vi "Get density continuous samples to func glob PN.vi"(0 "Timing SW trigger":tag="Dev1/port2/line7", 1 "Counter":tag="Dev1/ctr0", 2 "Device":tag="Dev1") -> ()   [LabVIEW 2011]
uses:
  <vilib>/Platform/TimedLoop/XDataNode/timing_clust.ctl
  <vilib>/Platform/TimedLoop/XDataNode/nitl_modes.ctl
  <vilib>/Platform/TimedLoop/XDataNode/wakeup.ctl
  <vilib>/DAQmx/read.llb/DAQmx Read (Digital Bool 1Line 1Point).vi
  <vilib>/DAQmx/read.llb/DAQmx Read (Counter U32 1Chan 1Samp).vi
  <vilib>/DAQmx/create/channels.llb/DAQmx Create Channel (DI-Digital Input).vi
  <vilib>/DAQmx/create/channels.llb/DAQmx Create Channel (CI-Count Edges).vi
  <vilib>/DAQmx/miscellaneous.llb/DAQmx Fill In Error Info.vi
  <vilib>/Platform/TimedLoop/XDataNode/XDataNode.xnode
  <vilib>/Platform/TimedLoop/XDataNode/XDNodeRunTimeDep.lvlib
panel:
  out "Density (kg/m^3)":dbl
  out "Sample DateTime":timestamp
  out "current sample":i32
  out "Density history":u32(graph)=997
  in  "stop":bool
  out "reset state":bool
  out "Error":errorcluster
  # "by Paul Nathan,06/03/2012"
  # "Revisions:\nDate       Desc.      Auth.\nx               x               x"
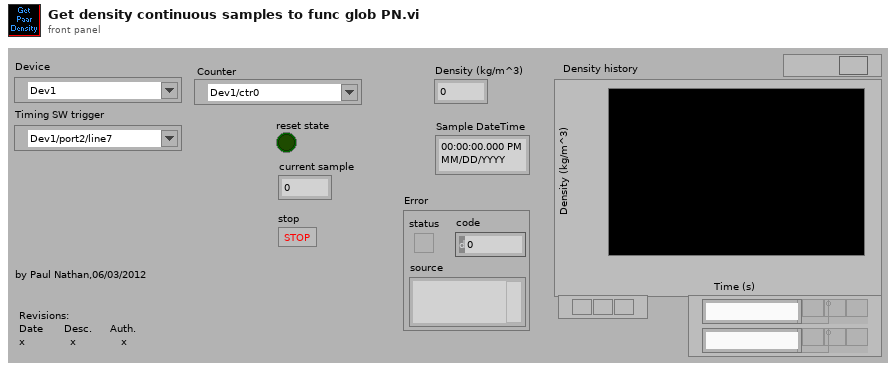
[diagram p1: front panel]
types:
  T1 = typedef "XDNodeRunTimeDep.lvlib/timing_clust.ctl" = cluster{"Expected End [f-1]":u64, "Actual End [f-1]":u64, "Finished Late? [f-1]":bool, "Expected End [i-1]":u64, "Actual End [i-1]":u64, "Finished Late? [i-1]":bool, "Expected Start [i]":u64, "Actual Start [i]":u64, "Expected Start [f]":u64, "Actual Start [f]":u64, "Source Name":string, "Structure Name":string, "Period":i64, "Deadline":i64, "Offset":i64, "Start":i64, "Priority":i32, "Timeout":i32, "Mode":T2, "Wakeup Reason":T3, "Error":errorcluster, "Source Type":string, "Secondary Source Type":string, "Global End Time":u64, "Global Start Time":u64, "Frame Duration":u64, "Iteration Duration":u64, "Assigned CPU":i32, "I/O Scan Engine Mode":u32}
  T2 = typedef "XDNodeRunTimeDep.lvlib/nitl_modes.ctl" = enum32{"No Change", "Process missed periods, maintain original phase", "Discard missed periods, maintain original phase", "Process missed periods, ignore original phase", "Discard missed periods, ignore original phase"}
  T3 = typedef "XDNodeRunTimeDep.lvlib/wakeup.ctl" = enum32{"Normal", "Aborted", "Asynchronous wakeup", "Timing source error", "Timed loop error", "Timeout"}
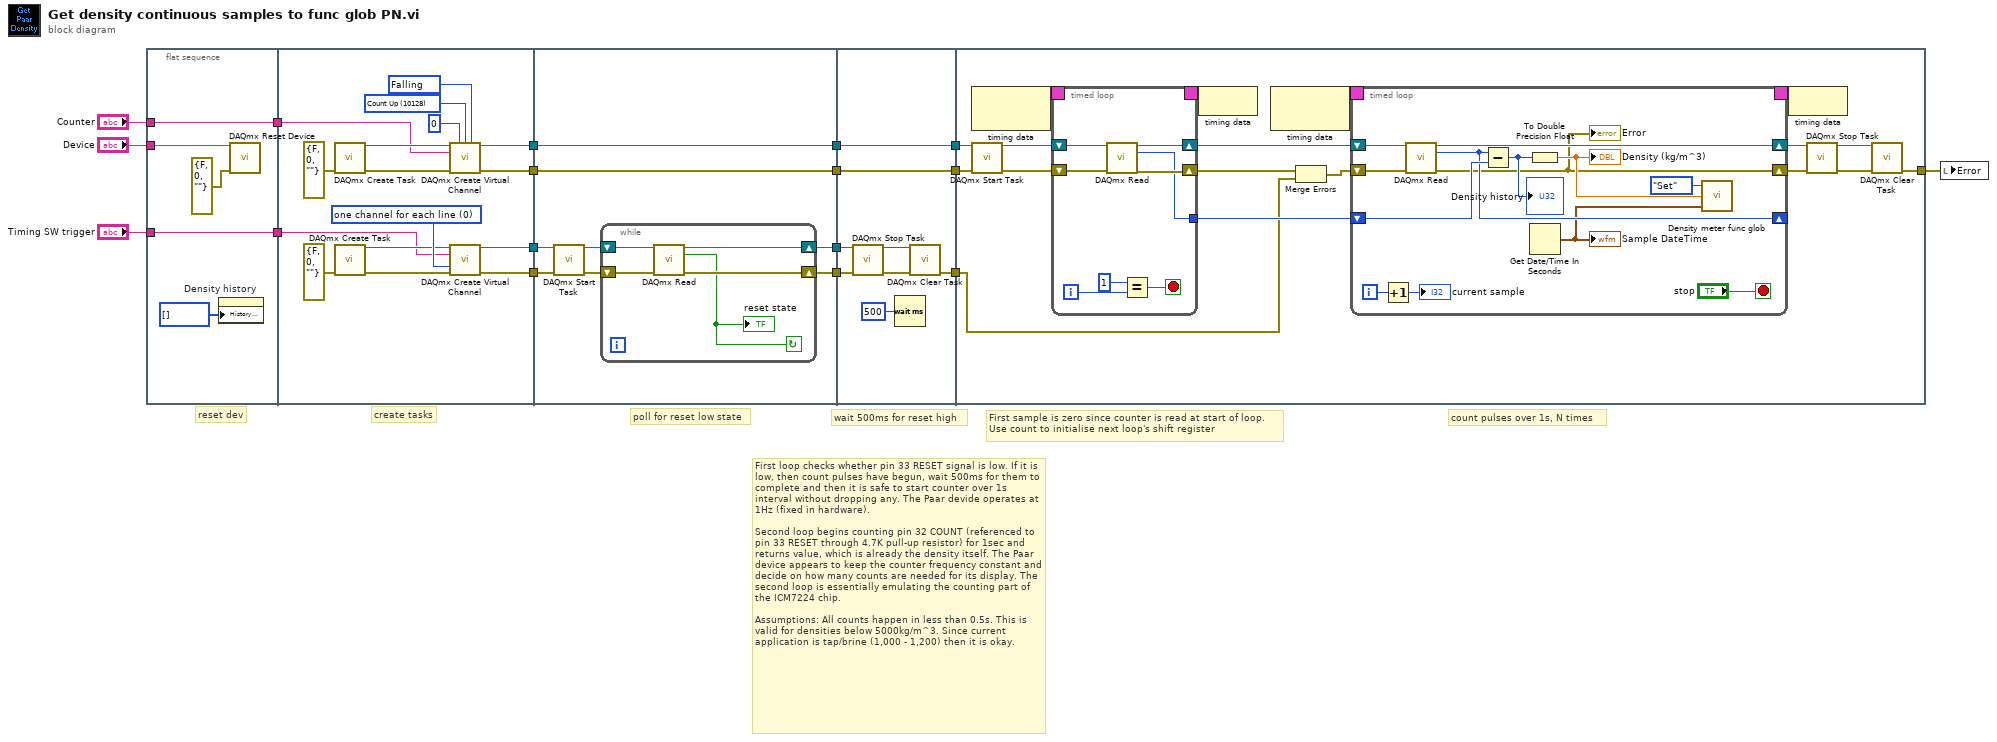
[diagram p0: block diagram]
diagram:
  # "First sample is zero since counter is read at start of loop.\nUse count to initialise next loop's shift register"
  # "count pulses over 1s, N times"
  # "wait 500ms for reset high"
  # "poll for reset low state"
  # "create tasks"
  # "reset dev"
  # "First loop checks whether pin 33 RESET signal is low. If it is low, then count pulses have begun, wait 500ms for them to complete and then it is safe to start counter over 1s interval without dropping any. The Paar devide operates at 1Hz (fixed in hardware).\n\nSecond loop begins counting pin 32 COUNT (referenced to pin 33 RESET through 4.7K pull-up resistor) for 1sec and returns value, which is already the density itself. The Paar device appears to keep the counter frequency constant and decide on how many counts are needed for its display. The second loop is essentially emulating the counting part of the ICM7224 chip.\n\nAssumptions: All counts happen in less than 0.5s. This is valid for densities below 5000kg/m^3. Since current application is tap/brine (1,000 - 1,200) then it is okay."
  n1 = flat-sequence {
    tunnel: [w21] -> w14
    tunnel: "Timing SW trigger" -> [w21]
    tunnel: [w20] -> w12
    tunnel: "Counter" -> [w20]
    tunnel: "Device" -> [w19]
    tunnel: w14 -> [w30]
    tunnel: w12 -> [w29]
    tunnel: [w25] -> w8
    tunnel: [w26] -> w6
    tunnel: [w24] -> w3
    tunnel: [w23] -> w2
    tunnel: [w46] -> w17
    tunnel: [w45] -> w16
    tunnel: [w44] -> w9
    tunnel: w8 -> [w44]
    tunnel: [w43] -> w7
    tunnel: w6 -> [w43]
    tunnel: w3 -> [w40]
    tunnel: w2 -> [w39]
    tunnel: w17 -> [w56]
    tunnel: w16 -> [w55]
    tunnel: [w54] -> w15
    tunnel: w9 -> [w53]
    tunnel: w7 -> [w52]
    tunnel: [w53] -> w5
    tunnel: [w52] -> w4
    tunnel: w15 -> [w63]
    tunnel: w5 -> [w71]
    tunnel: w4 -> [w70]
    tunnel: [w60] -> w1
    frame #0 {
      n2 = property on="Density history" class="WFChart (strict)"("History Data"=u32[] []) -> ()  [unwired: 2 in, 2 out]
      n3 = call <vilib>:"DAQmx Reset Device.vi"("device in"=w19, "error in"=errorcluster {"status"=FALSE, "code"=0, "source"=""}) -> ()  [unwired: 13 in, 1 out]
    }
    frame #1 {
      w34 = 10171 items=["Rising"=10280, "Falling"=10171] ("edge")
      w35 = 10128 items=["Count Up"=10128, "Count Down"=10124, "Externally Controlled"=10326] ("count direction")
      w32 = 0 items=["one channel for each line", "one channel for all lines"] ("line grouping")
      n4 = call <vilib>:"DAQmx Create Task.vi"("error in"=errorcluster {"status"=FALSE, "code"=0, "source"=""}) -> ("task out"=w37:refnum<k21>, "error out"=w38:errorcluster)  [unwired: 13 in]
      n5 = call <vilib>:"DAQmx Create Task.vi"("error in"=errorcluster {"status"=FALSE, "code"=0, "source"=""}) -> ("task out"=w31:refnum<k21>, "error out"=w33:errorcluster)  [unwired: 13 in]
      n6 = call-poly <vilib>:"DAQmx Create Virtual Channel.vi"("task in"=w37, "initial count"=u32 0, "count direction"=w35, "edge"=w34, "counter"=w29, "error in"=w38) -> ("task out"=w26:refnum<k21>, "error out"=w25:errorcluster)  [unwired: 8 in]
      n7 = call-poly <vilib>:"DAQmx Create Virtual Channel.vi"("task in"=w31, "lines"=w30, "line grouping"=w32, "error in"=w33) -> ("task out"=w23:refnum<k21>, "error out"=w24:errorcluster)  [unwired: 10 in]
    }
    frame #2 {
      n8 = call <vilib>:"DAQmx Start Task.vi"("task/channels in"=w39, "error in"=w40) -> ("task out"=w42:refnum<k21>, "error out"=w41:errorcluster)  [unwired: 12 in]
      n9 = while {
        shift-right: [w50] -> w45
        shift-left: w41 -> [w49]
        shift-right: [w48] -> w46
        shift-left: w42 -> [w51]
        stop <- w47 continue-if-true
        n10 = call-poly <vilib>:"DAQmx Read.vi"("task/channels in"=w51, "error in"=w49) -> ("task out"=w48:refnum<k21>, "data"=w47:bool, "error out"=w50:errorcluster)  [unwired: 11 in]
        "reset state" <- w47
      }
    }
    frame #3 {
      n11 = call <vilib>:"DAQmx Stop Task.vi"("task/channels in"=w56, "error in"=w55) -> ("task out"=w57:refnum<k21>, "error out"=w58:errorcluster)  [unwired: 12 in]
      n12 = Wait (ms)(milliseconds to wait=u32 500) -> ()  [unwired: 1 out]
      n13 = call <vilib>:"DAQmx Clear Task.vi"("task in"=w57, "error in"=w58) -> ("error out"=w54:errorcluster)  [unwired: 13 in]
    }
    frame #4 {
      n14 = node-c288() -> (w69:T1)  [unwired: 1 in]
      n15 = call <vilib>:"DAQmx Start Task.vi"("task/channels in"=w70, "error in"=w71) -> ("task out"=w66:refnum<k21>, "error out"=w65:errorcluster)  [unwired: 12 in]
      n16 = timed-loop {
        shift-right: [w83] -> w64
        shift-left: w66 -> [w84]
        shift-right: [w82] -> w62
        shift-left: w65 -> [w85]
        timing: w69 -> [_]
        timing-out: [_] -> w68
        tunnel: [w78] -> w67
        i -> [w81]
        stop <- w79 stop-if-true
        n17 = call-poly <vilib>:"DAQmx Read.vi"("task/channels in"=w84, "error in"=w85) -> ("task out"=w83:refnum<k21>, "data"=w78:u32, "error out"=w82:errorcluster)  [unwired: 11 in]
        n18 = Equal?(x=1 ("data"), y=w81) -> (x = y?=w79:bool)
      }
      n19 = node-c288(w68) -> ()
      n20 = node-c288() -> (w77:T1)  [unwired: 1 in]
      n21 = Merge Errors(w62, w63) -> (w61:errorcluster)
      n22 = timed-loop {
        shift-right: [w100] -> w73
        shift-left: w64 -> [w101]
        shift-right: [w90] -> w72
        shift-left: w61 -> [w102]
        timing: w77 -> [_]
        timing-out: [_] -> w76
        shift-right: [w97] -> _
        shift-left: w67 -> [w98]
        i -> [w99]
        stop <- "stop" stop-if-true
        n23 = Increment(x=w99) -> (x+1=→"current sample":i32)
        n24 = call-poly <vilib>:"DAQmx Read.vi"("task/channels in"=w101, "error in"=w102) -> ("task out"=w100:refnum<k21>, "data"=w97:u32, "error out"=w90:errorcluster)  [unwired: 11 in]
        "Error" <- w90
        n25 = Subtract(x=w97, y=w98) -> (x-y=w95:u32)
        "Density history" <- w95
        n26 = To Double Precision Float(number=w95) -> (double precision float=w93:dbl)
        "Density (kg/m^3)" <- w93
        n27 = Get Date/Time In Seconds() -> (seconds since 1Jan1904=w92:timestamp)
        "Sample DateTime" <- w92
        n28 = call "Density meter func glob.vi"("Sample DateTime in"=w92, "Density in"=w93, "Action"=enum16{"Get", "Set"}."Set") -> ()  [unwired: 2 out]
      }
      n29 = node-c288(w76) -> ()
      n30 = call <vilib>:"DAQmx Stop Task.vi"("task/channels in"=w73, "error in"=w72) -> ("task out"=w74:refnum<k21>, "error out"=w75:errorcluster)  [unwired: 12 in]
      n31 = call <vilib>:"DAQmx Clear Task.vi"("task in"=w74, "error in"=w75) -> ("error out"=w60:errorcluster)  [unwired: 13 in]
    }
  }
  n32 = local write "Error"(w1) -> ()
